vi "Cam Y.vi"() -> ()   [LabVIEW 2016]
panel:
  out "Cam Y":dbl
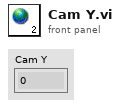
[diagram p1: front panel]
diagram:
